vi "RampVoltagewithDDSV15.vi"() -> ()   [LabVIEW 2016]
uses:
  <vilib>/DAQmx/write.llb/DAQmx Write (Digital 1D Wfm NChan NSamp).vi
  <vilib>/DAQmx/write.llb/DAQmx Write (Analog 2D DBL NChan NSamp).vi
  <vilib>/DAQmx/create/channels.llb/DAQmx Create Channel (AO-Voltage-Basic).vi
  <vilib>/DAQmx/create/channels.llb/DAQmx Create Channel (DO-Digital Output).vi
  <vilib>/DAQmx/configure/timing.llb/DAQmx Timing (Sample Clock).vi
  <vilib>/DAQmx/configure/trigger.llb/DAQmx Start Trigger (Digital Edge).vi
  <vilib>/Waveform/DWDTOps.llb/DWDT Boolean Array to Digital.vi
  <vilib>/Waveform/DWDTOps.llb/DWDT Uncompress Digital.vi
  <vilib>/DAQmx/miscellaneous.llb/DAQmx Fill In Error Info.vi
  <vilib>/Waveform/DTblOps.llb/DTbl Digital to Analog.vi
  <resource>/objmgr/daqmx.rc
  <vilib>/Utility/file.llb/Write Delimited Spreadsheet (DBL).vi
panel:
  out "ao3 Samples":i32=2001
  in  "DDS Trig High Time (ms)":dbl=2.0 step=0.01
  out "ao0 Samples":i32=2001
  in  "Ramp 2 Amplitude":dbl=0.4
  in  "Ramp 4 Amplitude":dbl=0.4
  in  "Ramp 3 Amplitude":dbl=0.4
  in  "Ramp 1 Amplitude":dbl=0.4
  in  "Ramp 4 Duration (ms)":dbl=0.2
  in  "Plateau 2 (ms)":dbl=1.6
  in  "Ramp 3 Duration (ms)":dbl=0.2
  in  "Delay 2 (ms)":dbl=2.0
  in  "Ramp 2 Duration (ms)":dbl=0.2
  in  "Plateau 1 (ms)":dbl=1.6
  in  "Ramp 1 Duration (ms)":dbl=0.2
  in  "Delay 1 (ms)":dbl=1.0
  out "ao2 Samples":i32=2001
  in  "ao2  File Path":path=path "C:/Users/Plexal_Machine/Documents/MM2toDDS/DDS VIs/Example1.txt"
  in  "Phase Lock Switch\n(TTL High - Lock Off)":bool=TRUE
  in  "Phase Lock Switch (Port 0 Line 1)":tag="Dev2/port0/line1"
  out "Digital Output":cluster{i32, dbl, dbl[][]}(graph)={0, 1e-05, [[0.0, 0.0, 0.0, 0.0, 0.0, 0.0, 0.0, 0.0, 0.0, 0.0, 0.0, 0.0, 0.0, 0.0, 0.0, 0.0, 0.0, 0.0, 0.0, 0.0, 0.0, 0.0, 0.0, 0.0, 0.0, 0.0, 0.0, 0.0, 0.0, 0.0, 0.0, 0.0, 0.0, 0.0, 0.0, 0.0, 0.0, 0.0, 0.0, 0.0, 0.0, 0.0, 0.0, 0.0, 0.0, 0.0, 0.0, 0.0, 0.0, 0.0, 0.0, 0.0, 0.0, 0.0, 0.0, 0.0, 0.0, 0.0, 0.0, 0.0, 0.0, 0.0, 0.0, 0.0, 0.0, 0.0, 0.0, 0.0, 0.0, 0.0, 0.0, 0.0, 0.0, 0.0, 0.0, 0.0, 0.0, 0.0, 0.0, 0.0, 0.0, 0.0, 0.0, 0.0, 0.0, 0.0, 0.0, 0.0, 0.0, 0.0, 0.0, 0.0, 0.0, 0.0, 0.0, 0.0, 0.0, 0.0, 0.0, 0.0, 0.0, 0.0, 0.0, 0.0, 0.0, 0.0, 0.0, 0.0, 0.0, 0.0, 0.0, 0.0, 0.0, 0.0, 0.0, 0.0, 0.0, 0.0, 0.0, 0.0, 0.0, 0.0, 0.0, 5.0, 5.0, 5.0, 5.0, 5.0, 5.0, 5.0, 5.0, 5.0, 5.0, 5.0, 5.0, 5.0, 5.0, 5.0, 5.0, 5.0, 5.0, 5.0, 5.0, 5.0, 5.0, 5.0, 5.0, 5.0, 5.0, 5.0, 5.0, 5.0, 5.0, 5.0, 5.0, 5.0, 5.0, 5.0, 5.0, 5.0, 5.0, 5.0, 5.0, 5.0, 5.0, 5.0, 5.0, 5.0, 5.0, 5.0, 5.0, 5.0, 5.0, 5.0, 5.0, 5.0, 5.0, 5.0, 5.0, 5.0, 5.0, 5.0, 5.0, 5.0, 5.0, 5.0, 5.0, 5.0, 5.0, 5.0, 5.0, 5.0, 5.0, 5.0, 5.0, 5.0, 5.0, 5.0, 5.0, 5.0, 5.0, 5.0, 5.0, 5.0, 5.0, 5.0, 5.0, 5.0, 5.0, 5.0, 5.0, 5.0, 5.0, 5.0, 5.0, 5.0, 5.0, 5.0, 5.0, 5.0, 5.0, 5.0, 5.0, 5.0, 5.0, 5.0, 5.0, 5.0, 5.0, 5.0, 5.0, 5.0, 5.0, 5.0, 5.0, 5.0, 5.0, 5.0, 5.0, 5.0, 5.0, 5.0, 5.0, 5.0, 5.0, 5.0, 5.0, 5.0, 5.0, 5.0, 5.0, 5.0, 5.0, 5.0, 5.0, 5.0, 5.0, 5.0, 5.0, 5.0, 5.0, 5.0, 5.0, 5.0, 5.0, 5.0, 5.0, 5.0, 5.0, 5.0, 5.0, 5.0, 5.0, 5.0, 5.0, 5.0, 5.0, 5.0, 5.0, 5.0, 5.0, 5.0, 5.0, 5.0, 5.0, 5.0, 5.0, 5.0, 5.0, 5.0, 5.0, 5.0, 5.0, 5.0, 5.0, 5.0, 5.0, 5.0, 5.0, 5.0, 5.0, 5.0, 5.0, 5.0, 5.0, 5.0, 5.0, 5.0, 5.0, 5.0, 5.0, 5.0, 5.0, 5.0, 5.0, 5.0, 5.0, 5.0, 5.0, 5.0, 5.0, 5.0, 5.0, 5.0, 5.0, 5.0, 5.0, 5.0, 5.0, 5.0, 5.0, 5.0, 5.0, 5.0, 5.0, 5.0, 5.0, 5.0, 5.0, 5.0, 5.0, 5.0, 5.0, 5.0, 5.0, 5.0, 5.0, 5.0, 5.0, 5.0, 5.0, 5.0, 5.0, 5.0, 5.0, 5.0, 5.0, 5.0, 5.0, 5.0, 5.0, 5.0, 5.0, 5.0, 5.0, 5.0, 5.0, 5.0, 5.0, 5.0, 5.0, 5.0, 5.0, 5.0, 5.0, 5.0, 5.0, 5.0, 5.0, 5.0, 5.0, 5.0, 5.0, 5.0, 5.0, 5.0, 5.0, 5.0, 5.0, 5.0, 5.0, 5.0, 5.0, 5.0, 5.0, 5.0, 5.0, 5.0, 5.0, 5.0, 5.0, 5.0, 5.0, 5.0, 5.0, 5.0, 5.0, 5.0, 5.0, 5.0, 5.0, 5.0, 5.0, 5.0, 5.0, 5.0, 5.0, 5.0, 5.0, 5.0, 5.0, 5.0, 5.0, 5.0, 5.0, 5.0, 5.0, 5.0, 5.0, 5.0, 5.0, 5.0, 5.0, 5.0, 5.0, 5.0, 5.0, 5.0, 5.0, 5.0, 5.0, 5.0, 5.0, 5.0, 5.0, 5.0, 5.0, 5.0, 5.0, 5.0, 5.0, 5.0, 5.0, 5.0, 5.0, 5.0, 5.0, 5.0, 5.0, 5.0, 5.0, 5.0, 5.0, 5.0, 5.0, 5.0, 5.0, 5.0, 5.0, 5.0, 5.0, 5.0, 5.0, 5.0, 5.0, 5.0, 5.0, 5.0, 5.0, 5.0, 5.0, 5.0, 5.0, 5.0, 5.0, 5.0, 5.0, 5.0, 5.0, 5.0, 5.0, 5.0, 5.0, 5.0, 5.0, 5.0, 5.0, 5.0, 5.0, 5.0, 5.0, 5.0, 5.0, 5.0, 5.0, 5.0, 5.0, 5.0, 5.0, 5.0, 5.0, 5.0, 5.0, 5.0, 5.0, 5.0, 5.0, 5.0, 5.0, 5.0, 5.0, 5.0, 5.0, 0.0, 0.0, 0.0, 0.0, 0.0, 0.0, 0.0, 0.0, 0.0, 0.0, 0.0, 0.0, 0.0, 0.0, 0.0, 0.0, 0.0, 0.0, 0.0, 0.0, 0.0, 0.0, 0.0, 0.0, 0.0, 0.0, 0.0, 0.0, 0.0, 0.0, 0.0, 0.0, 0.0, 0.0, 0.0, 0.0, 0.0, 0.0, 0.0, 0.0, 0.0, 0.0, 0.0, 0.0, 0.0, 0.0, 0.0, 0.0, 0.0, 0.0, 0.0, 0.0, 0.0, 0.0, 0.0, 0.0, 0.0, 0.0, 0.0, 0.0, 0.0, 0.0, 0.0, 0.0, 0.0, 0.0, 0.0, 0.0, 0.0, 0.0, 0.0, 0.0, 0.0, 0.0, 0.0, 0.0, 0.0, 0.0, 0.0, 0.0, 0.0, 0.0, 0.0, 0.0, 0.0, 0.0, 0.0, 0.0, 0.0, 0.0, 0.0, 0.0, 0.0, 0.0, 0.0, 0.0, 0.0, 0.0, 0.0, 0.0, 0.0, 0.0, 0.0, 0.0, 0.0, 0.0, 0.0, 0.0, 0.0, 0.0, 0.0, 0.0, 0.0, 0.0, 0.0, 0.0, 0.0, 0.0, 0.0, 0.0, 0.0, 0.0, 0.0, 0.0, 0.0, 0.0, 0.0, 0.0, 0.0, 0.0, 0.0, 0.0, 0.0, 0.0, 0.0, 0.0, 0.0, 0.0, 0.0, 0.0, 0.0, 0.0, 0.0, 0.0, 0.0, 0.0, 0.0, 0.0, 0.0, 0.0, 0.0, 0.0, 0.0, 0.0, 0.0, 0.0, 0.0, 0.0, 0.0, 0.0, 0.0, 0.0, 0.0, 0.0, 0.0, 0.0, 0.0, 0.0, 0.0, 0.0, 0.0, 0.0, 0.0, 0.0, 0.0, 0.0, 0.0, 0.0, 0.0, 0.0, 0.0, 0.0, 0.0, 0.0, 0.0, 0.0, 0.0, 0.0, 0.0, 0.0, 0.0, 0.0, 0.0, 0.0, 0.0, 0.0, 0.0, 0.0, 0.0, 0.0, 0.0, 0.0, 0.0, 0.0, 0.0, 0.0, 0.0, 0.0, 0.0, 0.0, 0.0, 0.0, 0.0, 0.0, 0.0, 0.0, 0.0, 0.0, 0.0, 0.0, 0.0, 0.0, 0.0, 0.0, 0.0, 0.0, 0.0, 0.0, 0.0, 0.0, 0.0, 0.0, 0.0, 0.0, 0.0, 0.0, 0.0, 0.0, 0.0, 0.0, 0.0, 0.0, 0.0, 0.0, 0.0, 0.0, 0.0, 0.0, 0.0, 0.0, 0.0, 0.0, 0.0, 0.0, 0.0, 0.0, 0.0, 0.0, 0.0, 0.0, 0.0, 0.0, 0.0, 0.0, 0.0, 0.0, 0.0, 0.0, 0.0, 0.0, 0.0, 0.0, 0.0, 0.0, 0.0, 0.0, 0.0, 0.0], [5.0, 5.0, 5.0, 5.0, 5.0, 5.0, 5.0, 5.0, 5.0, 5.0, 5.0, 5.0, 5.0, 5.0, 5.0, 5.0, 5.0, 5.0, 5.0, 5.0, 5.0, 5.0, 5.0, 5.0, 5.0, 5.0, 5.0, 5.0, 5.0, 5.0, 5.0, 5.0, 5.0, 5.0, 5.0, 5.0, 5.0, 5.0, 5.0, 5.0, 5.0, 5.0, 5.0, 5.0, 5.0, 5.0, 5.0, 5.0, 5.0, 5.0, 5.0, 5.0, 5.0, 5.0, 5.0, 5.0, 5.0, 5.0, 5.0, 5.0, 5.0, 5.0, 5.0, 5.0, 5.0, 5.0, 5.0, 5.0, 5.0, 5.0, 5.0, 5.0, 5.0, 5.0, 5.0, 5.0, 5.0, 5.0, 5.0, 5.0, 5.0, 5.0, 5.0, 5.0, 5.0, 5.0, 5.0, 5.0, 5.0, 5.0, 5.0, 5.0, 5.0, 5.0, 5.0, 5.0, 5.0, 5.0, 5.0, 5.0, 5.0, 5.0, 5.0, 5.0, 5.0, 5.0, 5.0, 5.0, 5.0, 5.0, 5.0, 5.0, 5.0, 5.0, 5.0, 5.0, 5.0, 5.0, 5.0, 5.0, 5.0, 5.0, 5.0, 5.0, 5.0, 5.0, 5.0, 5.0, 5.0, 5.0, 5.0, 5.0, 5.0, 5.0, 5.0, 5.0, 5.0, 5.0, 5.0, 5.0, 5.0, 5.0, 5.0, 5.0, 5.0, 5.0, 5.0, 5.0, 5.0, 5.0, 5.0, 5.0, 5.0, 5.0, 5.0, 5.0, 5.0, 5.0, 5.0, 5.0, 5.0, 5.0, 5.0, 5.0, 5.0, 5.0, 5.0, 5.0, 5.0, 5.0, 5.0, 5.0, 5.0, 5.0, 5.0, 5.0, 5.0, 5.0, 5.0, 5.0, 5.0, 5.0, 5.0, 5.0, 5.0, 5.0, 5.0, 5.0, 5.0, 5.0, 5.0, 5.0, 5.0, 5.0, 5.0, 5.0, 5.0, 5.0, 5.0, 5.0, 5.0, 5.0, 5.0, 5.0, 5.0, 5.0, 5.0, 5.0, 5.0, 5.0, 5.0, 5.0, 5.0, 5.0, 5.0, 5.0, 5.0, 5.0, 5.0, 5.0, 5.0, 5.0, 5.0, 5.0, 5.0, 5.0, 5.0, 5.0, 5.0, 5.0, 5.0, 5.0, 5.0, 5.0, 5.0, 5.0, 5.0, 5.0, 5.0, 5.0, 5.0, 5.0, 5.0, 5.0, 5.0, 5.0, 5.0, 5.0, 5.0, 5.0, 5.0, 5.0, 5.0, 5.0, 5.0, 5.0, 5.0, 5.0, 5.0, 5.0, 5.0, 5.0, 5.0, 5.0, 5.0, 5.0, 5.0, 5.0, 5.0, 5.0, 5.0, 5.0, 5.0, 5.0, 5.0, 5.0, 5.0, 5.0, 5.0, 5.0, 5.0, 5.0, 5.0, 5.0, 5.0, 5.0, 5.0, 5.0, 5.0, 5.0, 5.0, 5.0, 5.0, 5.0, 5.0, 5.0, 5.0, 5.0, 5.0, 5.0, 5.0, 5.0, 5.0, 5.0, 5.0, 5.0, 5.0, 5.0, 5.0, 5.0, 5.0, 5.0, 5.0, 5.0, 5.0, 5.0, 5.0, 5.0, 5.0, 5.0, 5.0, 5.0, 5.0, 5.0, 5.0, 5.0, 5.0, 5.0, 5.0, 5.0, 5.0, 5.0, 5.0, 5.0, 5.0, 5.0, 5.0, 5.0, 5.0, 5.0, 5.0, 5.0, 5.0, 5.0, 5.0, 5.0, 5.0, 5.0, 5.0, 5.0, 5.0, 5.0, 5.0, 5.0, 5.0, 5.0, 5.0, 5.0, 5.0, 5.0, 5.0, 5.0, 5.0, 5.0, 5.0, 5.0, 5.0, 5.0, 5.0, 5.0, 5.0, 5.0, 5.0, 5.0, 5.0, 5.0, 5.0, 5.0, 5.0, 5.0, 5.0, 5.0, 5.0, 5.0, 5.0, 5.0, 5.0, 5.0, 5.0, 5.0, 5.0, 5.0, 5.0, 5.0, 5.0, 5.0, 5.0, 5.0, 5.0, 5.0, 5.0, 5.0, 5.0, 5.0, 5.0, 5.0, 5.0, 5.0, 5.0, 5.0, 5.0, 5.0, 5.0, 5.0, 5.0, 5.0, 5.0, 5.0, 5.0, 5.0, 5.0, 5.0, 5.0, 5.0, 5.0, 5.0, 5.0, 5.0, 5.0, 5.0, 5.0, 5.0, 5.0, 5.0, 5.0, 5.0, 5.0, 5.0, 5.0, 5.0, 5.0, 5.0, 5.0, 5.0, 5.0, 5.0, 5.0, 5.0, 5.0, 5.0, 5.0, 5.0, 5.0, 5.0, 5.0, 5.0, 5.0, 5.0, 5.0, 5.0, 5.0, 5.0, 5.0, 5.0, 5.0, 5.0, 5.0, 5.0, 5.0, 5.0, 5.0, 5.0, 5.0, 5.0, 5.0, 5.0, 5.0, 5.0, 5.0, 5.0, 5.0, 5.0, 5.0, 5.0, 5.0, 5.0, 5.0, 5.0, 5.0, 5.0, 5.0, 5.0, 5.0, 5.0, 5.0, 5.0, 5.0, 5.0, 5.0, 5.0, 5.0, 5.0, 5.0, 5.0, 5.0, 5.0, 5.0, 5.0, 5.0, 5.0, 5.0, 5.0, 5.0, 5.0, 5.0, 5.0, 5.0, 5.0, 5.0, 5.0, 5.0, 5.0, 5.0, 5.0, 5.0, 5.0, 5.0, 5.0, 5.0, 5.0, 5.0, 5.0, 5.0, 5.0, 5.0, 5.0, 5.0, 5.0, 5.0, 5.0, 5.0, 5.0, 5.0, 5.0, 5.0, 5.0, 5.0, 5.0, 5.0, 5.0, 5.0, 5.0, 5.0, 5.0, 5.0, 5.0, 5.0, 5.0, 5.0, 5.0, 5.0, 5.0, 5.0, 5.0, 5.0, 5.0, 5.0, 5.0, 5.0, 5.0, 5.0, 5.0, 5.0, 5.0, 5.0, 5.0, 5.0, 5.0, 5.0, 5.0, 5.0, 5.0, 5.0, 5.0, 5.0, 5.0, 5.0, 5.0, 5.0, 5.0, 5.0, 5.0, 5.0, 5.0, 5.0, 5.0, 5.0, 5.0, 5.0, 5.0, 5.0, 5.0, 5.0, 5.0, 5.0, 5.0, 5.0, 5.0, 5.0, 5.0, 5.0, 5.0, 5.0, 5.0, 5.0, 5.0, 5.0, 5.0, 5.0, 5.0, 5.0, 5.0, 5.0, 5.0, 5.0, 5.0, 5.0, 5.0, 5.0, 5.0, 5.0, 5.0, 5.0, 5.0, 5.0, 5.0, 5.0, 5.0, 5.0, 5.0, 5.0, 5.0, 5.0, 5.0, 5.0, 5.0, 5.0, 5.0, 5.0, 5.0, 5.0, 5.0, 5.0, 5.0, 5.0, 5.0, 5.0, 5.0, 5.0, 5.0, 5.0, 5.0, 5.0, 5.0, 5.0, 5.0, 5.0, 5.0, 5.0, 5.0, 5.0, 5.0, 5.0, 5.0, 5.0, 5.0, 5.0, 5.0, 5.0, 5.0, 5.0, 5.0, 5.0, 5.0, 5.0, 5.0, 5.0, 5.0, 5.0, 5.0, 5.0, 5.0, 5.0, 5.0, 5.0, 5.0, 5.0, 5.0, 5.0, 5.0, 5.0, 5.0, 5.0, 5.0, 5.0, 5.0, 5.0, 5.0, 5.0, 5.0, 5.0, 5.0, 5.0, 5.0, 5.0, 5.0, 5.0, 5.0, 5.0, 5.0, 5.0, 5.0, 5.0, 5.0, 5.0, 5.0, 5.0, 5.0, 5.0, 5.0, 5.0, 5.0, 5.0, 5.0, 5.0, 5.0, 5.0, 5.0, 5.0, 5.0, 5.0, 5.0, 5.0, 5.0, 5.0, 5.0, 5.0, 5.0, 5.0, 5.0, 5.0, 5.0, 5.0, 5.0, 5.0, 5.0, 5.0, 5.0, 5.0, 5.0, 5.0, 5.0, 5.0, 5.0, 5.0, 5.0, 5.0, 5.0, 5.0, 5.0, 5.0, 5.0, 5.0, 5.0, 5.0, 5.0, 5.0, 5.0, 5.0, 5.0, 5.0, 5.0, 5.0, 5.0, 5.0, 5.0, 5.0, 5.0, 5.0, 5.0, 5.0, 5.0, 5.0, 5.0, 5.0, 5.0, 5.0, 5.0, 5.0, 5.0, 5.0]]}
  out "Analog Outputs":cluster{i32, dbl, dbl[][]}(graph)={0, 4e-06, array4x2001[8004 elements]}
  in  "DDS Trigger (Port 0 Line 0)":tag="Dev2/port0/line0"
  in  "DDS trigger delay (ms)":dbl=0.23 step=0.01
  in  "error in 2":errorcluster caption="error in"
  in  "ao1 ramp amplitude (V)":dbl=0.04
  in  "SolsTiS 2 - Fast Piezo (ao3)":tag="Dev2/ao3"
  in  "SolsTiS 2 - Slow Piezo (ao2)":tag="Dev2/ao2"
  in  "Trigger delay NI (ms)":dbl=1.0
  in  "Trigger Input (PFI0)":tag="/Dev2/PFI0"
  in  "SolsTiS 1 - Fast Piezo (ao1)":tag="Dev2/ao1"
  in  "SolsTiS 1 - Slow Piezo (ao0)":tag="Dev2/ao0"
  in  "Plateau duration (ms)":dbl=2.0 step=0.01
  in  "Ramp duration (ms)":dbl=2.0 step=0.01
  in  "ao0 ramp amplitude (V)":dbl=0.09 step=0.001
  in  "error in":errorcluster
  # "MAGIS LASER SYSTEM\nChirp Control"
  # "Ramp Definition"
  # "Output Monitor"
  # "Channel Definition"
  # "Fast Piezo (A03)"
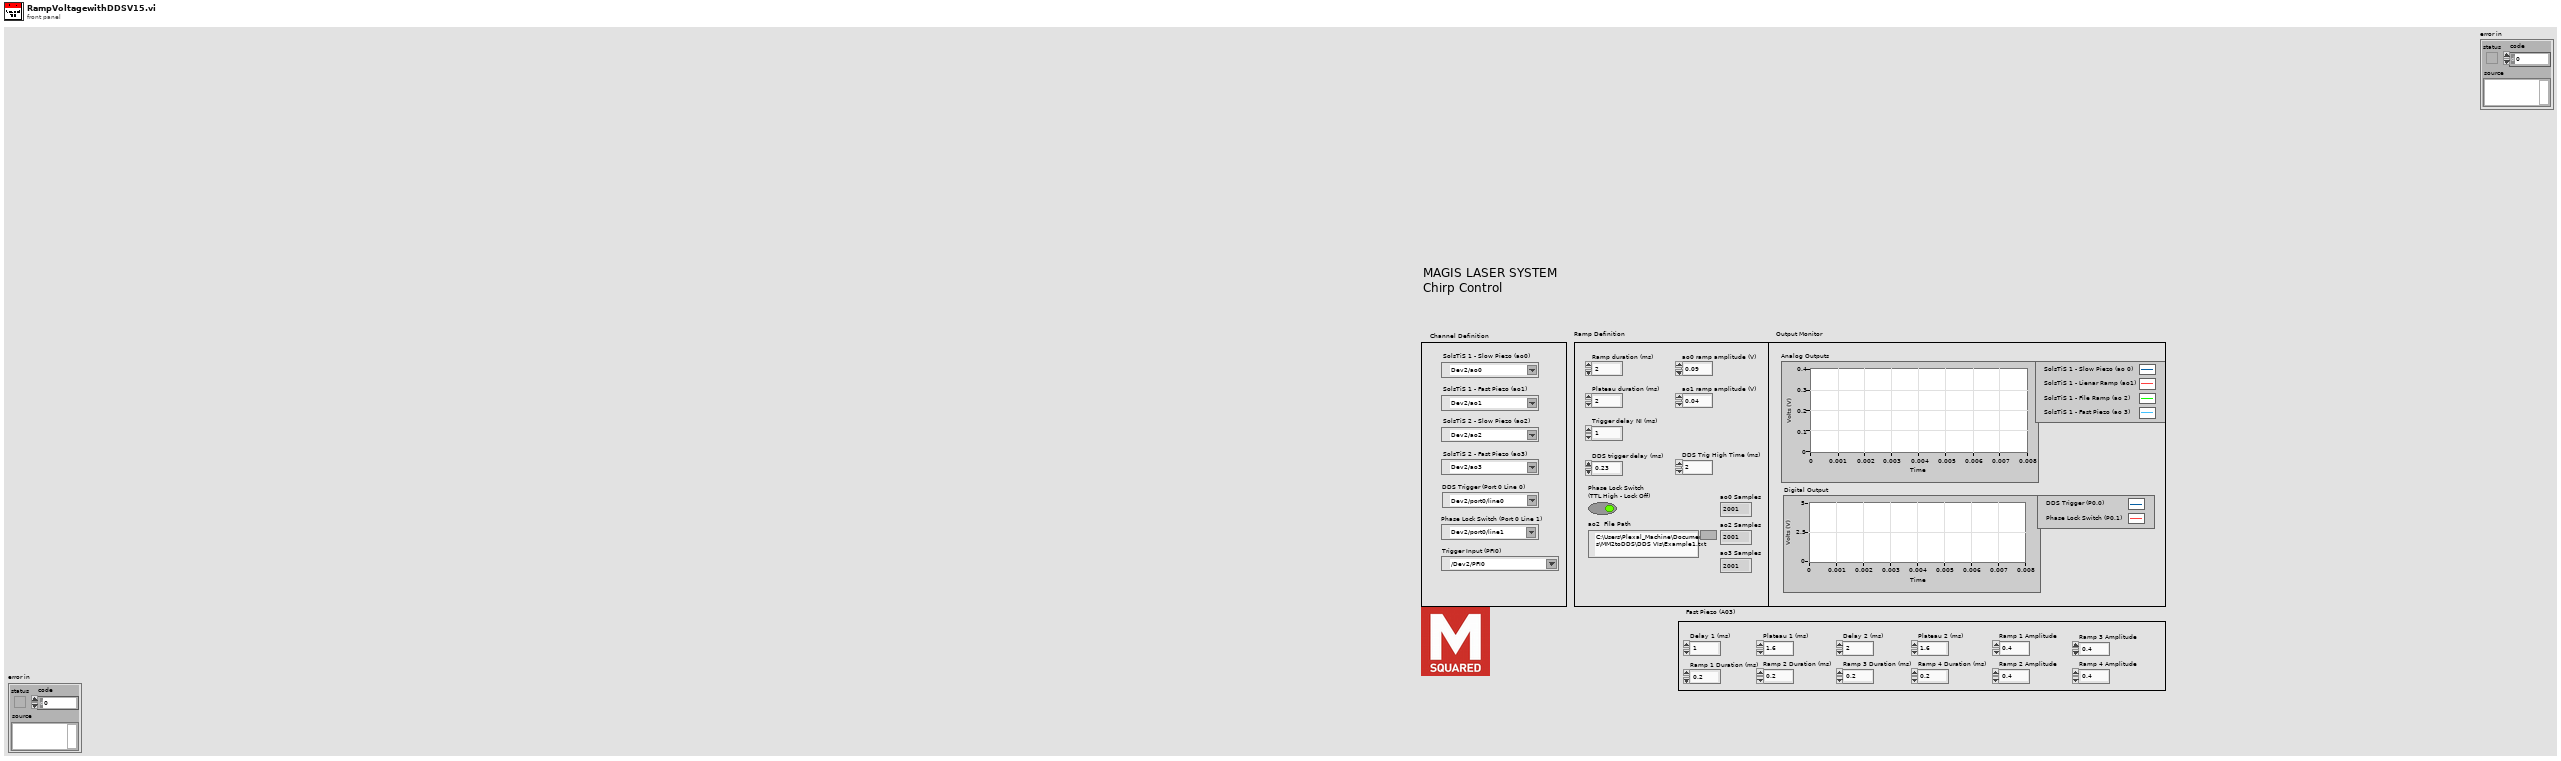
[diagram p1: front panel]
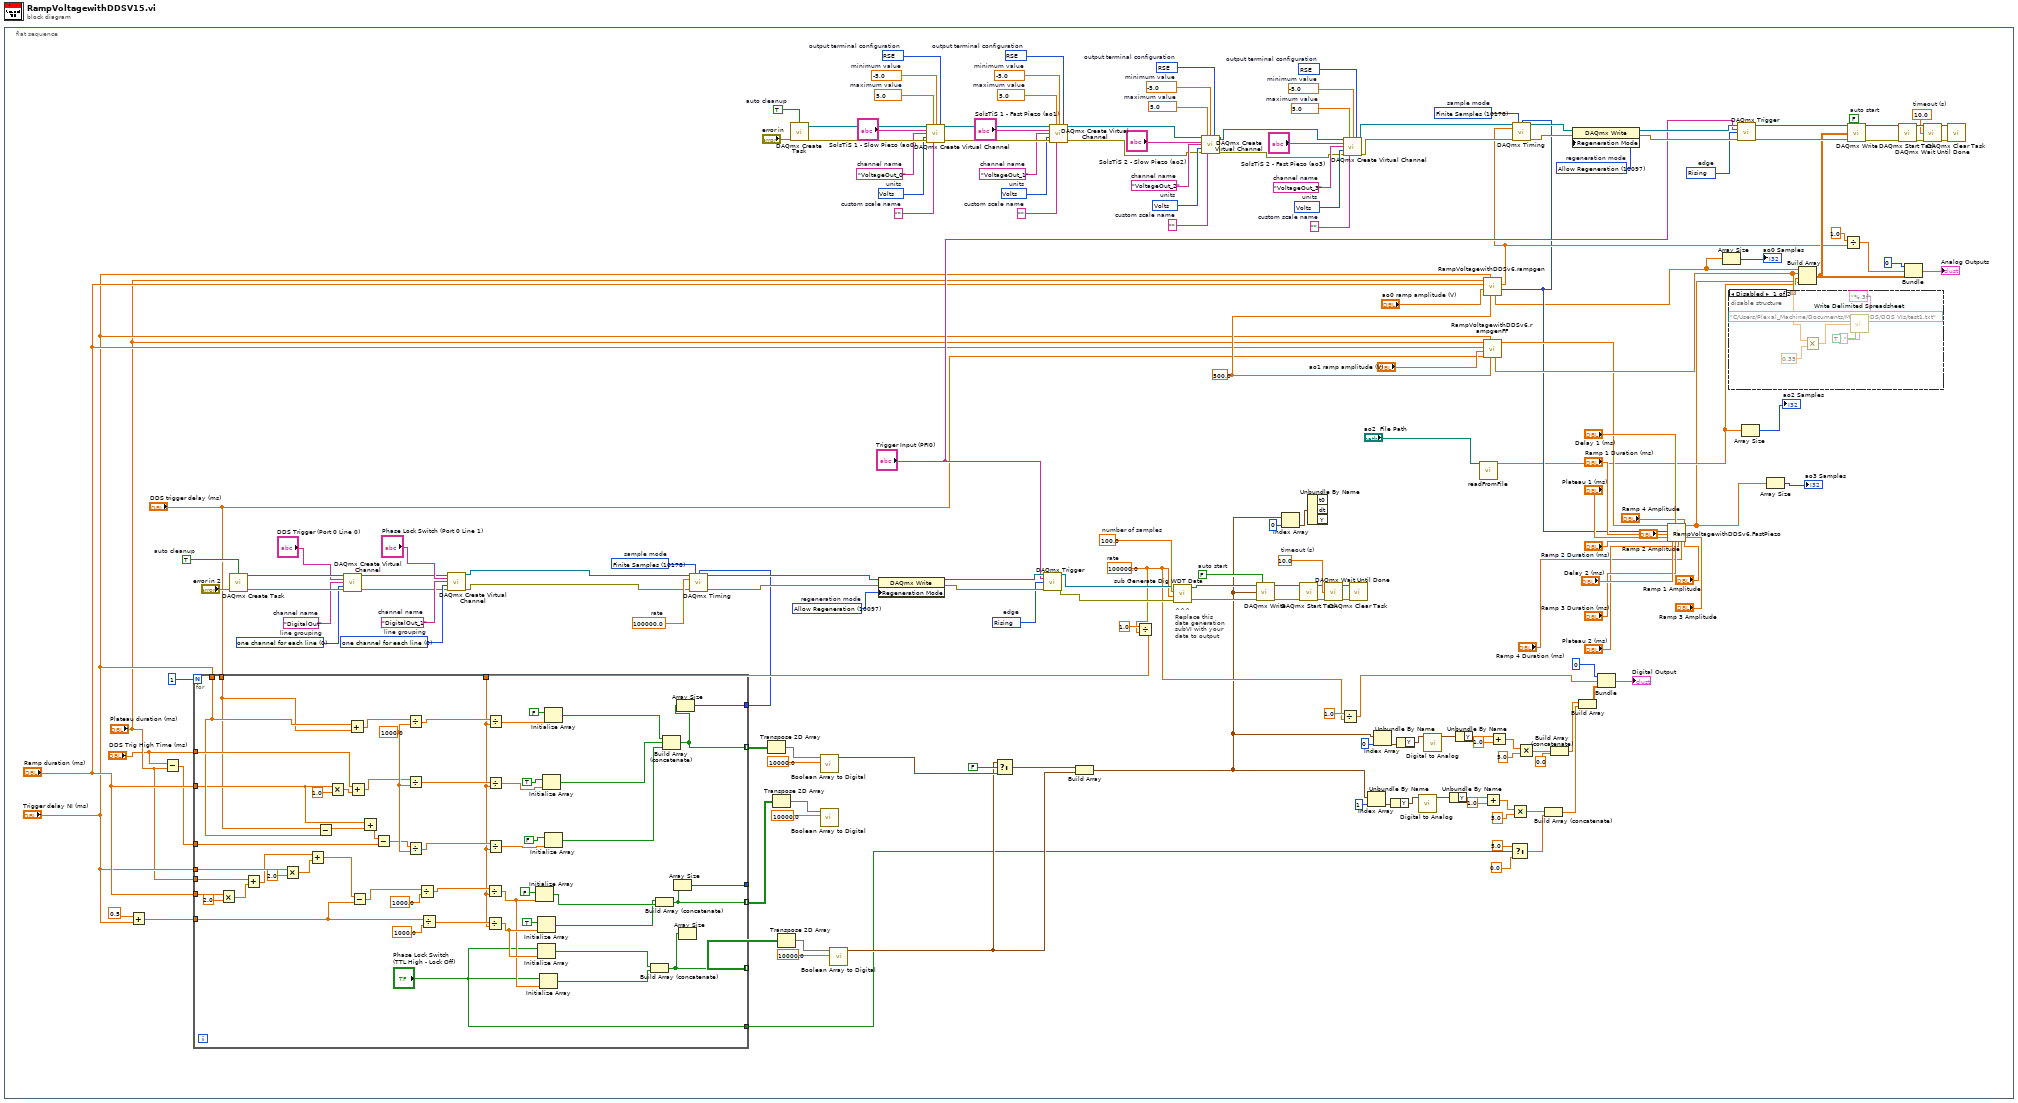
[diagram p0: block diagram]
diagram:
  n1 = flat-sequence {
    frame #0 {
      w4 = 10.0  # timeout (s)
      w8 = FALSE  # auto start
      w75 = 0 items=["one channel for each line", "one channel for all lines"]  # line grouping
      w74 = "DigitalOut_1"  # channel name
      w133 = 500.0 ("No of samples in ramp (500 or less)")
      w109 = 10280 items=["Rising"=10280, "Falling"=10171]  # edge
      w111 = 10097 items=["Allow Regeneration"=10097, "Do Not Allow Regeneration"=10158]  # regeneration mode
      w114 = 10178 items=["Finite Samples"=10178, "Continuous Samples"=10123, "Hardware Timed Single Point"=12522]  # sample mode
      w115 = 100000.0  # rate
      w118 = 0 items=["one channel for each line", "one channel for all lines"]  # line grouping
      w117 = "DigitalOut"  # channel name
      w120 = TRUE  # auto cleanup
      w131 = 10.0  # timeout (s)
      w83 = 100000.0  # rate
      w128 = 100.0  # number of samples
      w125 = FALSE  # auto start
      w139 = 10083 items=["Default"=-1, "RSE"=10083, "Differential"=10106, "Pseudodifferential"=12529]  # output terminal configuration
      w140 = 10348 items=["Volts"=10348, "From Custom Scale"=10065]  # units
      w141 = "VoltageOut_3"  # channel name
      w142 = ""  # custom scale name
      w143 = -5.0  # minimum value
      w144 = 5.0  # maximum value
      w148 = 10083 items=["Default"=-1, "RSE"=10083, "Differential"=10106, "Pseudodifferential"=12529]  # output terminal configuration
      w149 = 10348 items=["Volts"=10348, "From Custom Scale"=10065]  # units
      w150 = "VoltageOut_2"  # channel name
      w151 = ""  # custom scale name
      w152 = -5.0  # minimum value
      w153 = 5.0  # maximum value
      w159 = 10280 items=["Rising"=10280, "Falling"=10171]  # edge
      w161 = 10097 items=["Allow Regeneration"=10097, "Do Not Allow Regeneration"=10158]  # regeneration mode
      w164 = 10178 items=["Finite Samples"=10178, "Continuous Samples"=10123, "Hardware Timed Single Point"=12522]  # sample mode
      w166 = 10083 items=["Default"=-1, "RSE"=10083, "Differential"=10106, "Pseudodifferential"=12529]  # output terminal configuration
      w167 = 10348 items=["Volts"=10348, "From Custom Scale"=10065]  # units
      w168 = "VoltageOut_1"  # channel name
      w169 = ""  # custom scale name
      w170 = -5.0  # minimum value
      w171 = 5.0  # maximum value
      w173 = 10083 items=["Default"=-1, "RSE"=10083, "Differential"=10106, "Pseudodifferential"=12529]  # output terminal configuration
      w174 = 10348 items=["Volts"=10348, "From Custom Scale"=10065]  # units
      w175 = "VoltageOut_0"  # channel name
      w177 = ""  # custom scale name
      w178 = -5.0  # minimum value
      w179 = 5.0  # maximum value
      w181 = TRUE  # auto cleanup
      # "^^^\nReplace this\ndata generation\nsubVI with your\ndata to output"
      n2 = Add(x=0.5 ("DDS Trigger delay (ms)"), y="Trigger delay NI (ms)") -> (x+y=w69:dbl)
      n3 = Subtract(x="DDS Trig High Time (ms)", y="Plateau duration (ms)") -> (x-y=w17:dbl)
      n4 = call <vilib>:"DAQmx Create Task.vi"("auto cleanup"=w120, "error in"="error in 2") -> ("task out"=w119:refnum<k21>, "error out"=w121:errorcluster)  [unwired: 12 in]
      n5 = call-poly <vilib>:"DAQmx Create Virtual Channel.vi"("task in"=w119, "lines"="DDS Trigger (Port 0 Line 0)", "name to assign"=w117, "line grouping"=w118, "error in"=w121) -> ("task out"=w71:refnum<k21>, "error out"=w72:errorcluster)  [unwired: 9 in]
      n6 = call-poly <vilib>:"DAQmx Create Virtual Channel.vi"("task in"=w71, "lines"="Phase Lock Switch (Port 0 Line 1)", "name to assign"=w74, "line grouping"=w75, "error in"=w72) -> ("task out"=w48:refnum<k21>, "error out"=w47:errorcluster)  [unwired: 9 in]
      n7 = call <vilib>:"DAQmx Create Task.vi"("auto cleanup"=w181, "error in"="error in") -> ("task out"=w180:refnum<k21>, "error out"=w182:errorcluster)  [unwired: 12 in]
      n8 = call-poly <vilib>:"DAQmx Create Virtual Channel.vi"("task in"=w180, "maximum value"=w179, "minimum value"=w178, "output terminal configuration"=w173, "physical channels"="SolsTiS 1 - Slow Piezo (ao0)", "name to assign"=w175, "units"=w174, "error in"=w182, "custom scale name"=w177) -> ("task out"=w172:refnum<k21>, "error out"=w176:errorcluster)  [unwired: 5 in]
      n9 = call-poly <vilib>:"DAQmx Create Virtual Channel.vi"("task in"=w172, "maximum value"=w171, "minimum value"=w170, "output terminal configuration"=w166, "physical channels"="SolsTiS 1 - Fast Piezo (ao1)", "name to assign"=w168, "units"=w167, "error in"=w176, "custom scale name"=w169) -> ("task out"=w146:refnum<k21>, "error out"=w145:errorcluster)  [unwired: 5 in]
      n10 = Divide(x=1.0, y=w83) -> (x/y=w105:dbl)
      n11 = for {
        N: 1 -> [_]
        tunnel: w105 -> [w219]
        tunnel: [w234] -> w102 mode=indexing
        tunnel: [w233] -> w101
        tunnel: "Trigger delay NI (ms)" -> [w199]
        tunnel: w69 -> [w225]
        tunnel: "Ramp duration (ms)" -> [w229]
        tunnel: "Plateau duration (ms)" -> [w226]
        tunnel: [w216] -> _
        tunnel: "Trigger delay NI (ms)" -> [w213]
        tunnel: [w210] -> w66 mode=indexing
        tunnel: [w192] -> w63 mode=indexing
        tunnel: "Ramp duration (ms)" -> [w197]
        tunnel: "DDS Trig High Time (ms)" -> [w201]
        tunnel: ["Phase Lock Switch\n(TTL High - Lock Off)"] -> w44
        tunnel: "DDS trigger delay (ms)" -> [w195]
        tunnel: w17 -> [w191]
        w244 = 1000.0
        n12 = Multiply(x=w229, y=2.0) -> (x*y=w227:dbl)
        n13 = Add(x=w226, y=w227) -> (x+y=w212:dbl)
        n14 = Multiply(x=w213, y=2.0) -> (x*y=w214:dbl)
        n15 = Add(x=w212, y=w214) -> (x+y=w211:dbl)
        n16 = Subtract(x=w199, y=w195) -> (x-y=w196:dbl)
        n17 = Multiply(x=w197, y=1.0) -> (x*y=w202:dbl)
        n18 = Add(x=w199, y=w195) -> (x+y=w232:dbl)
        n19 = Add(x=w201, y=w202) -> (x+y=w200:dbl)
        n20 = Subtract(x=w211, y=w225) -> (x-y=w222:dbl)
        n21 = Add(x=w197, y=w196) -> (x+y=w194:dbl)
        n22 = Subtract(x=w194, y=w191) -> (x-y=w193:dbl)
        n23 = Divide(x=w232, y=w244) -> (x/y=w243:dbl)
        n24 = Divide(x=w200, y=w244) -> (x/y=w242:dbl)
        n25 = Divide(x=w193, y=w244) -> (x/y=w241:dbl)
        n26 = Divide(x=w222, y=1000.0) -> (x/y=w221:dbl)
        n27 = Divide(x=w225, y=1000.0) -> (x/y=w220:dbl)
        n28 = Divide(x=w221, y=w219) -> (x/y=w206:dbl)
        n29 = Divide(x=w220, y=w219) -> (x/y=w209:dbl)
        n30 = Divide(x=w243, y=w219) -> (x/y=w238:dbl)
        n31 = Divide(x=w242, y=w219) -> (x/y=w237:dbl)
        n32 = Divide(x=w241, y=w219) -> (x/y=w236:dbl)
        n33 = Initialize Array(FALSE, w206) -> (w218:bool[])
        n34 = Initialize Array(TRUE, w209) -> (w217:bool[])
        n35 = Initialize Array("Phase Lock Switch\n(TTL High - Lock Off)", w209) -> (w208:bool[])
        n36 = Initialize Array("Phase Lock Switch\n(TTL High - Lock Off)", w206) -> (w207:bool[])
        n37 = Initialize Array(TRUE, w237) -> (w205:bool[])
        n38 = Initialize Array(FALSE, w236) -> (w204:bool[])
        n39 = Initialize Array(FALSE, w238) -> (w235:bool[])
        n40 = Build Array (concatenate)(w208, w207) -> (w192:bool[])
        n41 = Build Array (concatenate)(w217, w218) -> (w210:bool[])
        n42 = Build Array (concatenate)(w235, w205, w204) -> (w234:bool[])
        n43 = Array Size(array=w210) -> (size(s)=w216:i32)
        n44 = Array Size(array=w234) -> (size(s)=w233:i32)
        n45 = Array Size(array=w192) -> ()  [unwired: 1 out]
      }
      n46 = call-poly <vilib>:"DAQmx Timing.vi"("task/channels in"=w48, "sample mode"=w114, "samples per channel"=w101, "rate"=w115, "error in"=w47) -> ("task out"=w113:refnum<k21>, "error out"=w116:errorcluster)  [unwired: 9 in]
      n47 = Transpose 2D Array(2D array=w102) -> (transposed array=w103:bool[][])
      n48 = Transpose 2D Array(2D array=w66) -> (transposed array=w67:bool[][])
      n49 = Transpose 2D Array(2D array=w63) -> (transposed array=w64:bool[][])
      n50 = call-poly <vilib>:"Boolean Array to Digital.vi"("sample rate"=10000.0, "boolean array"=w103) -> ("digital waveform"=w52:digitalwaveform)  [unwired: 8 in, 1 out]
      n51 = call-poly <vilib>:"Boolean Array to Digital.vi"("sample rate"=10000.0, "boolean array"=w67) -> ()  [unwired: 8 in, 2 out]
      n52 = call-poly <vilib>:"Boolean Array to Digital.vi"("sample rate"=10000.0, "boolean array"=w64) -> ("digital waveform"=w45:digitalwaveform)  [unwired: 8 in, 1 out]
      n53 = property class="DAQmx Write"(reference=w113, error in=w116, "Regeneration Mode"=w111) -> (reference out=w110:refnum<k21>, error out=w112:errorcluster)
      n54 = Select(t=w45, s=FALSE ("Constant PO.0?"), f=w52) -> (s? t:f=w50:digitalwaveform)
      n55 = call-poly <vilib>:"DAQmx Trigger.vi"("task/channels in"=w110, "source"="Trigger Input (PFI0)", "edge"=w109, "error in"=w112) -> ("task out"=w108:refnum<k21>, "error out"=w107:errorcluster)  [unwired: 10 in]
      n56 = Build Array(w50, w45) -> (w49:digitalwaveform[])
      n57 = call <vilib>:"sub Generate Dig WDT Data.vi"("task in"=w108, "number of samples"=w128, "update rate"=w83, "error in"=w107) -> ("task out"=w127:refnum<k21>, "error out"=w126:errorcluster)  [unwired: 1 in, 1 out]
      n58 = call-poly <vilib>:"DAQmx Create Virtual Channel.vi"("task in"=w146, "maximum value"=w153, "minimum value"=w152, "output terminal configuration"=w148, "physical channels"="SolsTiS 2 - Slow Piezo (ao2)", "name to assign"=w150, "units"=w149, "error in"=w145, "custom scale name"=w151) -> ("task out"=w137:refnum<k21>, "error out"=w136:errorcluster)  [unwired: 5 in]
      n59 = call-poly <vilib>:"DAQmx Write.vi"("task/channels in"=w127, "auto start"=w125, "data"=w49, "error in"=w126) -> ("task out"=w129:refnum<k21>, "error out"=w130:errorcluster)  [unwired: 9 in, 1 out]
      n60 = Index Array(array=w49, index=0) -> (element=w123:digitalwaveform)
      n61 = call <vilib>:"DAQmx Start Task.vi"("task/channels in"=w129, "error in"=w130) -> ("task out"=w9:refnum<k21>, "error out"=w10:errorcluster)  [unwired: 12 in]
      n62 = Unbundle By Name(w123) -> ()  [unwired: 3 out]
      n63 = call <vilib>:"DAQmx Wait Until Done.vi"("task/channels in"=w9, "timeout (sec)"=w131, "error in"=w10) -> ("task out"=w12:refnum<k21>, "error out"=w11:errorcluster)  [unwired: 11 in]
      n64 = Divide(x=1.0, y=w83) -> (x/y=w82:dbl)
      n65 = call-poly <vilib>:"DAQmx Create Virtual Channel.vi"("task in"=w137, "maximum value"=w144, "minimum value"=w143, "output terminal configuration"=w139, "physical channels"="SolsTiS 2 - Fast Piezo (ao3)", "name to assign"=w141, "units"=w140, "error in"=w136, "custom scale name"=w142) -> ("task out"=w134:refnum<k21>, "error out"=w135:errorcluster)  [unwired: 5 in]
      n66 = call <vilib>:"DAQmx Clear Task.vi"("task in"=w12, "error in"=w11) -> ()  [unwired: 13 in, 1 out]
      n67 = Index Array(array=w49, index=1) -> (element=w61:digitalwaveform)
      n68 = Index Array(array=w49, index=0) -> (element=w93:digitalwaveform)
      n69 = Unbundle By Name(w61) -> ("Y"=w60:digitaldata)
      n70 = Unbundle By Name(w93) -> ("Y"=w92:digitaldata)
      n71 = call-poly <vilib>:"Digital to Analog.vi"("digital table"=w60) -> ("analog waveform"=w59:waveform(dbl))  [unwired: 7 in, 3 out]
      n72 = call-poly <vilib>:"Digital to Analog.vi"("digital table"=w92) -> ("analog waveform"=w91:waveform(dbl))  [unwired: 7 in, 3 out]
      n73 = Unbundle By Name(w59) -> ("Y"=w57:dbl[])
      n74 = Unbundle By Name(w91) -> ("Y"=w80:dbl[])
      n75 = call "readFromFile.vi"("file path (dialog if empty)"="ao2  File Path") -> ("data"=w22:dbl[])  [unwired: 10 in]
      n76 = call "RampVoltagewithDDSv6,rampgen.vi"("No of samples in ramp"=w133, "Trigger delay NI (ms)"="Trigger delay NI (ms)", "Ramp Amplitude (V)}"="ao0 ramp amplitude (V)", "Ramp duration (ms)"="Ramp duration (ms)", "Plateau duration (ms)"="Plateau duration (ms)") -> ("Numeric 2"=w25:i32, "Numeric"=w86:dbl, "Array"=w18:dbl[])  [unwired: 3 in, 1 out]
      n77 = call "RampVoltagewithDDSv6,rampgenFF.vi"("No of samples in ramp"=w133, "Trigger delay NI (ms)"="Trigger delay NI (ms)", "DDS Trigger Delay (ms)"="DDS trigger delay (ms)", "Ramp Amplitude (V)}"="ao1 ramp amplitude (V)", "Ramp duration (ms)"="Ramp duration (ms)", "Plateau duration (ms)"="Plateau duration (ms)") -> ("Sample rate"=w26:dbl, "Array"=w38:dbl[])  [unwired: 2 in, 2 out]
      n78 = Add(x=w57, y=1.0) -> (x+y=w56:dbl[])
      n79 = Add(x=w80, y=1.0) -> (x+y=w79:dbl[])
      n80 = Select(t=5.0, s=w44, f=0.0 ("y")) -> (s? t:f=w41:dbl)
      n81 = Multiply(x=w56, y=5.0) -> (x*y=w54:dbl[])
      n82 = call-poly <vilib>:"DAQmx Timing.vi"("task/channels in"=w134, "sample mode"=w164, "samples per channel"=w25, "rate"=w86, "error in"=w135) -> ("task out"=w163:refnum<k21>, "error out"=w165:errorcluster)  [unwired: 9 in]
      n83 = Multiply(x=w79, y=5.0) -> (x*y=w77:dbl[])
      n84 = Build Array (concatenate)(w54, w41) -> (w53:dbl[])
      n85 = Build Array (concatenate)(w77, 0.0 ("y")) -> (w76:dbl[])
      n86 = property class="DAQmx Write"(reference=w163, error in=w165, "Regeneration Mode"=w161) -> (reference out=w160:refnum<k21>, error out=w162:errorcluster)
      n87 = Build Array(w76, w53) -> (w88:dbl[][])
      n88 = Bundle(0, w82, w88) -> (→"Digital Output":cluster{i32, dbl, dbl[][]})  [unwired: 1 in]
      n89 = call "RampVoltagewithDDSv6,FastPiezo.vi"("Sample rate"=w26, "Ramp Samples"=w25, "Ramp 1 Duration (ms)"="Ramp 1 Duration (ms)", "Plateau 1 (ms)"="Plateau 1 (ms)", "Ramp 2 Duration (ms)"="Ramp 2 Duration (ms)", "Delay 2 (ms)"="Delay 2 (ms)", "Delay 1 (ms)"="Delay 1 (ms)", "Ramp 3 Duration (ms)"="Ramp 3 Duration (ms)", "Plateau 2 (ms)"="Plateau 2 (ms)", "Ramp 4 Duration (ms)"="Ramp 4 Duration (ms)", "Ramp 4 Amplitude"="Ramp 4 Amplitude", "Ramp 2 Amplitude"="Ramp 2 Amplitude", "Ramp 3 Amplitude"="Ramp 3 Amplitude", "Ramp 1 Amplitude"="Ramp 1 Amplitude") -> ("appended array"=w21:dbl[])  [unwired: 5 in]
      n90 = Array Size(array=w18) -> (size(s)=→"ao0 Samples":i32)
      n91 = disable-structure shown="Disabled" {
        disable-tunnel: w38 -> [w186 _]
        frame Disabled {
          n92 = Multiply(x=w186, y=0.35 ("x")) -> (x*y=w184:dbl[])
          n93 = call-poly <vilib>:"Write Delimited Spreadsheet.vi"("file path (dialog if empty)"=path "C:/Users/Plexal_Machine/Documents/MM2toDDS/DDS VIs/test1.txt", "format (%.3f)"="%.3f", "1D data"=w184, "transpose? (no:F)"=TRUE, "delimiter (\\t)"="," ("delimiter (\\t)")) -> ()  [unwired: 9 in, 2 out]
        }
        frame Enabled {
        }
      }
      n94 = call-poly <vilib>:"DAQmx Trigger.vi"("task/channels in"=w160, "source"="Trigger Input (PFI0)", "edge"=w159, "error in"=w162) -> ("task out"=w157:refnum<k21>, "error out"=w156:errorcluster)  [unwired: 10 in]
      n95 = Array Size(array=w22) -> (size(s)=→"ao2 Samples":i32)
      n96 = Array Size(array=w21) -> (size(s)=→"ao3 Samples":i32)
      n97 = Build Array(w18, w38, w22, w21) -> (w97:dbl[][])
      n98 = Divide(x=1.0, y=w86) -> (x/y=w85:dbl)
      n99 = call-poly <vilib>:"DAQmx Write.vi"("task/channels in"=w157, "auto start"=w8, "data"=w97, "error in"=w156) -> ("task out"=w3:refnum<k21>, "error out"=w2:errorcluster)  [unwired: 9 in, 1 out]
      n100 = call <vilib>:"DAQmx Start Task.vi"("task/channels in"=w3, "error in"=w2) -> ("task out"=w7:refnum<k21>, "error out"=w6:errorcluster)  [unwired: 12 in]
      n101 = Bundle(0, w85, w97) -> (→"Analog Outputs":cluster{i32, dbl, dbl[][]})  [unwired: 1 in]
      n102 = call <vilib>:"DAQmx Wait Until Done.vi"("task/channels in"=w7, "timeout (sec)"=w4, "error in"=w6) -> ("task out"=w1:refnum<k21>, "error out"=w5:errorcluster)  [unwired: 11 in]
      n103 = call <vilib>:"DAQmx Clear Task.vi"("task in"=w1, "error in"=w5) -> ()  [unwired: 13 in, 1 out]
    }
  }
